vi "PTSequencer.save settings.vi"(0 "i ref in":refnum<vi>, 2 "path":string, 3 "ms timeout (10000)":i32=10000, 5 "error in (no error)":errorcluster) -> (14 "i ref out":refnum<vi>, 17 "timed out":bool, 19 "error out":errorcluster)   [LabVIEW 2014, in "PTSequencer.lvlib"]
uses:
  PTSequencer.lvlib
  <vilib>/Utility/xml.llb/Write to XML File(string).vi
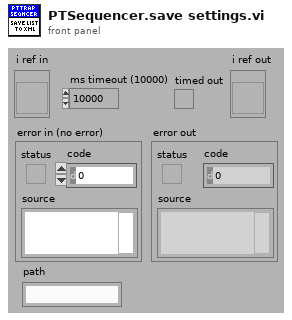
[diagram p1: front panel]
types:
  T1 = typedef "PTSequencer.lvlib/PTSequencer.i attribute.ctl" = cluster{"subsequence":bool, "mode":T2, "i step":i32, "nofLoops":i32, "i loop":i32, "Running":bool, "Paused":bool, "step done":bool, "loop done":bool, "seq done":bool, "DIM IDs":cluster{"step done":i32, "loop done":i32, "seq done":i32, "i step":i32, "i loop":i32}, "use stop conditions":bool, "stop conditions":T3[], "Step List":T5[], "DIM subsriptions":string[], "stop cond indexes":i32[], "step cond indexes":cluster{"step condition IDs":cluster{"step ID":i32, "condition ID":i32}[]}[], "Delay Start Time":timestamp, "status":string, "stopping":bool}
  T2 = typedef "PTSequencer.lvlib/PTSequencer.mode.ctl" = enum16{"single", "loop", "for loop"}
  T3 = typedef "PTSequencer.lvlib/PTSequencer.DIM service condition.ctl" = cluster{"DIM service":string, "descr":string, "nomValue":T4, "actValue":T4, "matched":bool, "DIM Status":cluster{"no link":bool, "quality":i32, "Time Stamp":timestamp}}
  T4 = typedef "CoreDefs.rawDataType.ctl" = i8[]
  T5 = typedef "PTSequencer.lvlib/PTSequencer.step.ctl" = cluster{"description":string, "object parameters":cluster{"object":string, "selector":string, "descriptor":string, "data":T4, "subsequence":bool, "call mode":enum16{"Simple DIM", "Synchronous"}, "data in":T4}, "result action":cluster{"check":bool, "passed":enum16{"Next", "Previous", "Repeat", "Jump"}, "failed":enum16{"Next", "Previous", "Repeat", "Jump"}, "jumpID_passed":i32, "jumpID_failed":i32}, "conditions":T3[], "fulfilled ":bool, "use delay":bool, "delay time (s)":dbl, "ID":i32}
  T6 = cluster{"use stop conditions":bool, "stop conditions":T3[], "Step List":T5[]}
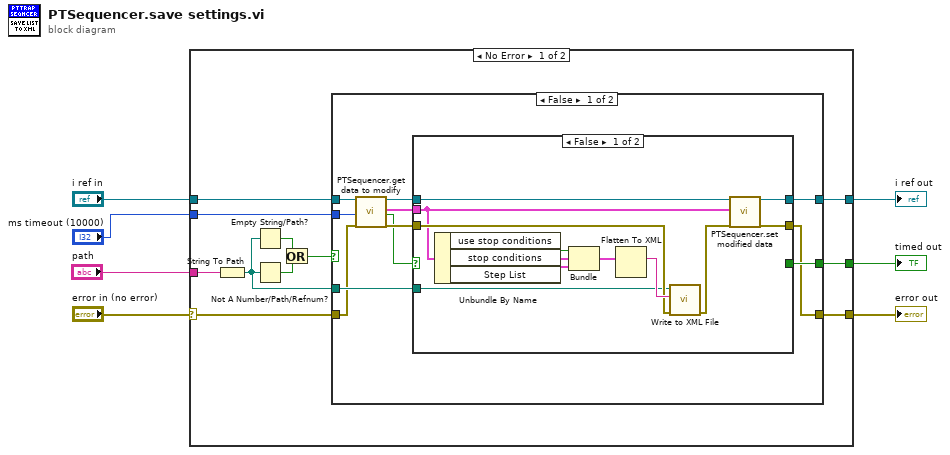
[diagram p0: block diagram]
diagram:
  n1 = case shown="No Error" "error in (no error)" {
    selector: "error in (no error)" -> [w9 w47]
    tunnel: "i ref in" -> [w18 w48]
    tunnel: [w16 w48] -> w5
    tunnel: [w8 w47] -> w4
    tunnel: "ms timeout (10000)" -> [w17 _]
    tunnel: [w15 _] -> w2
    tunnel: "path" -> [w14 _]
    frame No Error {
      n2 = String To Path(string=w14) -> (path=w10:path)
      n3 = Empty String/Path?(string/path=w10) -> (empty?=w13:bool)
      n4 = Not A Number/Path/Refnum?(number/path/refnum=w10) -> (NaN/Path/Refnum?=w12:bool)
      n5 = Or(x=w13, y=w12) -> (x .or. y?=w11:bool)
      n6 = case shown="False" w11 {
        tunnel: w18 -> [w29 w45]
        tunnel: w17 -> [w24 _]
        tunnel: [w23 w45] -> w16
        tunnel: [w22 _] -> w15
        tunnel: w10 -> [w21 _]
        tunnel: w9 -> [w20 w46]
        tunnel: [w19 w46] -> w8
        frame False {
          n7 = call "PTSequencer.get data to modify.vi"("i ref in"=w29, "ms timeout (10000)"=w24, "error in (no error)"=w20) -> ("i ref out"=w28:refnum<vi>, "i attribute"=w26:T1, "timed out"=w25:bool, "error out"=w27:errorcluster)  [unwired: 13 in]
          n8 = case shown="False" w25 {
            selector: w25 -> [_ w42]
            tunnel: w28 -> [w41 w44]
            tunnel: w27 -> [w35 w43]
            tunnel: w26 -> [w30 _]
            tunnel: [w32 w44] -> w23
            tunnel: [w33 w43] -> w19
            tunnel: [_ w42] -> w22
            tunnel: w21 -> [w31 _]
            frame False {
              n9 = Unbundle By Name(w30) -> ("use stop conditions"=w39:bool, "stop conditions"=w38:T3[], "Step List"=w37:T5[])
              n10 = Bundle("use stop conditions"=w39, "stop conditions"=w38, "Step List"=w37) -> (w36:T6)  [unwired: 1 in]
              n11 = Flatten To XML(anything=w36) -> (xml string=w40:string)
              n12 = call-poly <vilib>:"Write to XML File.vi"("error in (no error)"=w35, "XML Input"=w40, "XML File Path"=w31) -> ("error out"=w34:errorcluster)  [unwired: 6 in, 2 out]
              n13 = call "PTSequencer.set modified data.vi"("i ref in"=w41, "CLASS.i attribute"=w30, "error in (no error)"=w34) -> ("i ref out"=w32:refnum<vi>, "error out"=w33:errorcluster)  [unwired: 15 in]
            }
            frame True {
            }
          }
        }
        frame True {
        }
      }
    }
    frame Error {
    }
  }
  "error out" <- w4
  "i ref out" <- w5
  "timed out" <- w2
